vi "set_chunk_time_interval.vi"(7 "connection_reference":T1, 8 "error in (no error)":errorcluster, 10 "chunk_time_interval":dbl=86400.0 format="%<%H:%M:%S>t", 11 "hyper_table_name":string) -> (0 "error out":errorcluster)   [LabVIEW 2015, in "lv-timescaledb.lvlib"]
uses:
  lv-timescaledb.lvlib
  <vilib>/addons/database/Connection.llb/Conn ObjectReference.ctl
  <vilib>/addons/database/Command.llb/Cmd Execute.vi
  <vilib>/addons/database/Recordset.llb/Rec Destroy - Command.vi
  <vilib>/addons/database/Command.llb/Cmd Delete.vi
  <vilib>/addons/database/NI_Database_API.lvlib
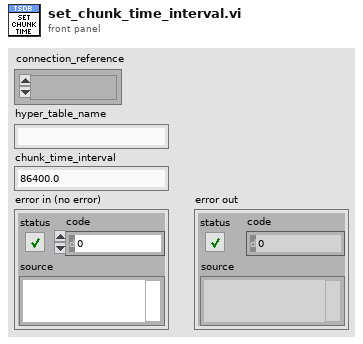
[diagram p1: front panel]
types:
  T1 = typedef "NI_Database_API.lvlib/Conn ObjectReference.ctl" = refnum<k1>
  T2 = cluster{"hyper_table_name":string, "interval":string}
  T3 = typedef "NI_Database_API.lvlib/DB Tools Parameter Info.ctl" = cluster{"parameter name":string, "type":T4, "direction":T5, "value":variant}
  T4 = typedef "NI_Database_API.lvlib/DB Tools DataTypes.ctl" = enum16{"String", "Long (I32)", "Single (SGL)", "Double (DBL)", "Date/Time", "Binary"}
  T5 = typedef "NI_Database_API.lvlib/DB Tools Parameter Dir.ctl" = enum32{"Input", "Output", "Input/Output", "Return Value"}
  T6 = typedef "NI_Database_API.lvlib/Cmd ObjectReference.ctl" = refnum<k1>
  T7 = typedef "NI_Database_API.lvlib/Cmd-Rec Object Reference.ctl" = refnum<k1>
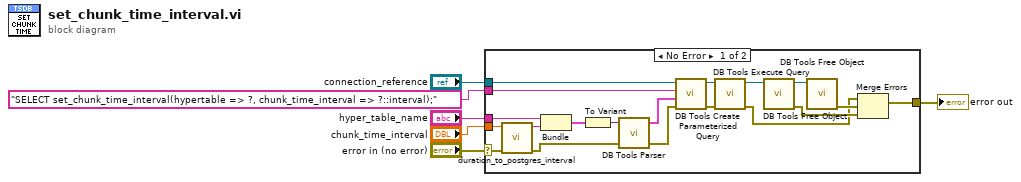
[diagram p0: block diagram]
diagram:
  n1 = case shown="No Error" "error in (no error)" {
    selector: "error in (no error)" -> [w10 w26]
    tunnel: "hyper_table_name" -> [w15 _]
    tunnel: "connection_reference" -> [w21 _]
    tunnel: [w25 w26] -> w2
    tunnel: "SELECT set_chunk_time_interval(hypertable => ?, chunk_time_interval => ?::interval);" -> [w20 _]
    tunnel: "chunk_time_interval" -> [w9 _]
    frame No Error {
      n2 = call "duration_to_postgres_interval.vi"("error in (no error)"=w10, "relative_time"=w9) -> ("error out"=w7:errorcluster, "interval"=w8:string)  [unwired: 8 in]
      n3 = Bundle("hyper_table_name"=w15, "interval"=w8) -> (w14:T2)  [unwired: 1 in]
      n4 = To Variant(anything=w14) -> (Variant=w13:variant)
      n5 = call <vilib>:"DB Tools Parser.vi"("error in (no error)"=w7, "variant"=w13) -> ("error out"=w18:errorcluster, "parameters"=w19:T3[])  [unwired: 2 in]
      n6 = call <vilib>:"DB Tools Create Parameterized Query.vi"("error in (no error)"=w18, "parameters"=w19, "SQL query"=w20, "connection reference"=w21) -> ("error out"=w22:errorcluster, "command reference"=w23:T6)  [unwired: 3 in, 1 out]
      n7 = call-poly <vilib>:"DB Tools Execute Query.vi"("error in (no error)"=w22, "command reference"=w23) -> ("error out"=w12:errorcluster, "command-recordset reference"=w11:T7)  [unwired: 6 in]
      n8 = call-poly <vilib>:"DB Tools Free Object.vi"("command-recordset reference"=w11) -> ("error out"=w16:errorcluster, "command reference"=w24:T6)  [unwired: 9 in]
      n9 = call-poly <vilib>:"DB Tools Free Object.vi"("command reference"=w24) -> ("error out"=w17:errorcluster)  [unwired: 9 in, 1 out]
      n10 = Merge Errors(w12, w17, w16) -> (w25:errorcluster)
    }
    frame Error {
    }
  }
  "error out" <- w2
